vi "addDevice.vi"(10 "Cluster":T1={"Simulator.Instance"=refnum, "Instance"=refnum, "Simulator"=refnum, "Nodes"={}, "Selected.Node"=refnum, "Properties"={}, "Selected.Property"=refnum, "Tree.Components.Ref"=refnum, "Tree.Properties.Ref"=refnum, "DisplayType"=enum."SYSTEM_OVERVIEW", "Readonly?"=[]}) -> (2 "Cluster 2":T1={"Simulator.Instance"=refnum, "Instance"=refnum, "Simulator"=refnum, "Nodes"={}, "Selected.Node"=refnum, "Properties"={}, "Selected.Property"=refnum, "Tree.Components.Ref"=refnum, "Tree.Properties.Ref"=refnum, "DisplayType"=enum."SYSTEM_OVERVIEW", "Readonly?"=[]})   [LabVIEW 2022 SP3, in "Property Editor.lvlib"]
uses:
  Property Editor.lvlib
  Public/Classes/IComponent/IComponent.lvclass
  TypeDef/Context.ctl
  TypeDef/DisplayType.ctl
  Public/Classes/IProperty/IProperty.lvclass
panel:
  in  "stop":bool
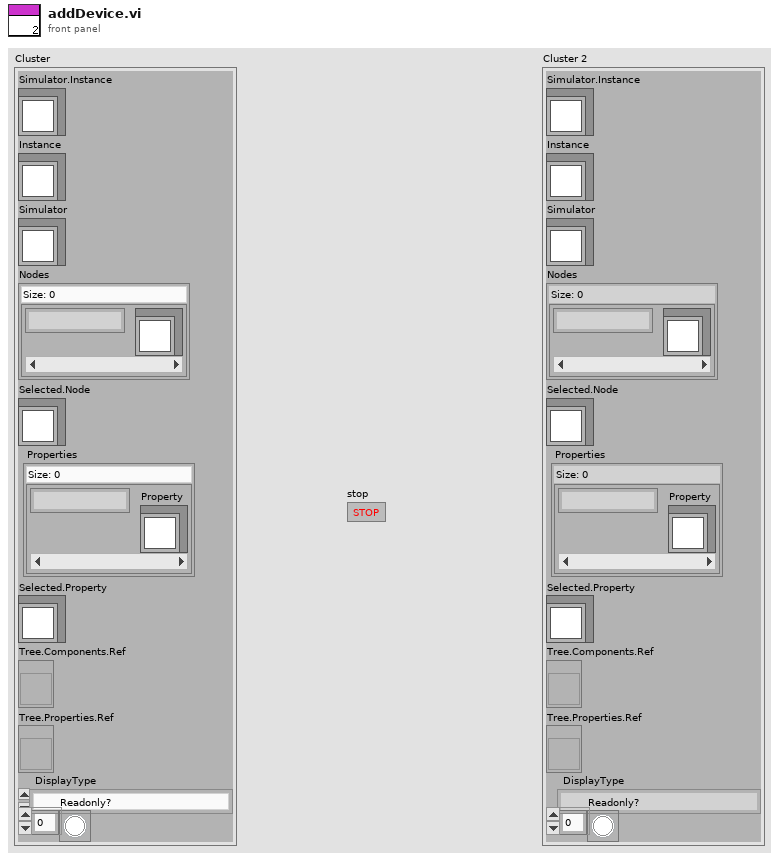
[diagram p1: front panel]
types:
  T1 = typedef "Property Editor.lvlib/Context.ctl" = cluster{"Simulator.Instance":refnum<class "IComponent.lvclass">, "Instance":refnum<class "IComponent.lvclass">, "Simulator":refnum<class "IComponent.lvclass">, "Nodes":map{string, refnum<class "IComponent.lvclass">}, "Selected.Node":refnum<class "IComponent.lvclass">, "Properties":map{string, refnum<class "IProperty.lvclass">}, "Selected.Property":refnum<class "IProperty.lvclass">, "Tree.Components.Ref":refnum<vi>, "Tree.Properties.Ref":refnum<vi>, "DisplayType":T2, "Readonly?":bool[]}
  T2 = typedef "Property Editor.lvlib/DisplayType.ctl" = enum16{"SYSTEM_OVERVIEW", "SIGNALS", "CHANNELS", "FUNCTION_BLOCKS", "TOPOLOGY", "TOPOLOGY_CUSTOM_COMPONENTS", "UNSPECIFIED"}
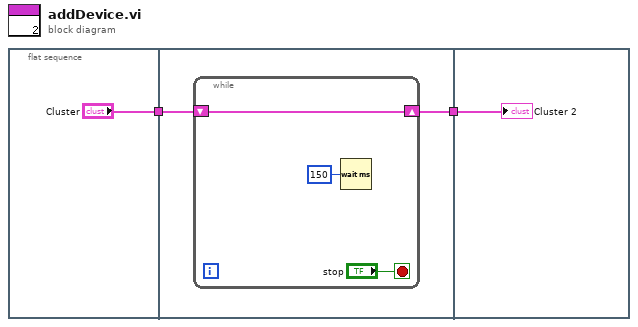
[diagram p0: block diagram]
diagram:
  n1 = flat-sequence {
    tunnel: ["Cluster"] -> w2
    tunnel: w2 -> [w5]
    tunnel: [w4] -> w1
    tunnel: w1 -> [w9]
    frame #0 {
    }
    frame #1 {
      n2 = while {
        shift-right: [w8] -> w4
        shift-left: w5 -> [w8]
        stop <- "stop" stop-if-true
        n3 = Wait (ms)(milliseconds to wait=u32 150) -> ()  [unwired: 1 out]
      }
    }
    frame #2 {
      "Cluster 2" <- w9
    }
  }
